vi "Copy Installed VIPM Files to Unpacked Data Folder.vi"(8 "error in (no error)":errorcluster, 9 "LabVIEW version":string, 10 "VIPM Package Installed Filepaths":path[](array[path]), 11 "Unpacked Data Folder":path) -> (0 "error out":errorcluster, 1 "LabVIEW version out":string)   [LabVIEW 2014, in "vipm-to-nipm-package-converter.lvlib"]
doc: "Copies the installed files of the specified VIPM package (.vip) into the corresponding nipkg folder structure\n\nINPUT(S):\n<b>LabVIEW version</b>: Specifies the LabVIEW version for the NIPM package to support (\"14.0\", \"14.0 (64-bit)\", \"18.0\", \"18.0 (64-bit)\", etc)"
uses:
  vipm-to-nipm-package-converter.lvlib
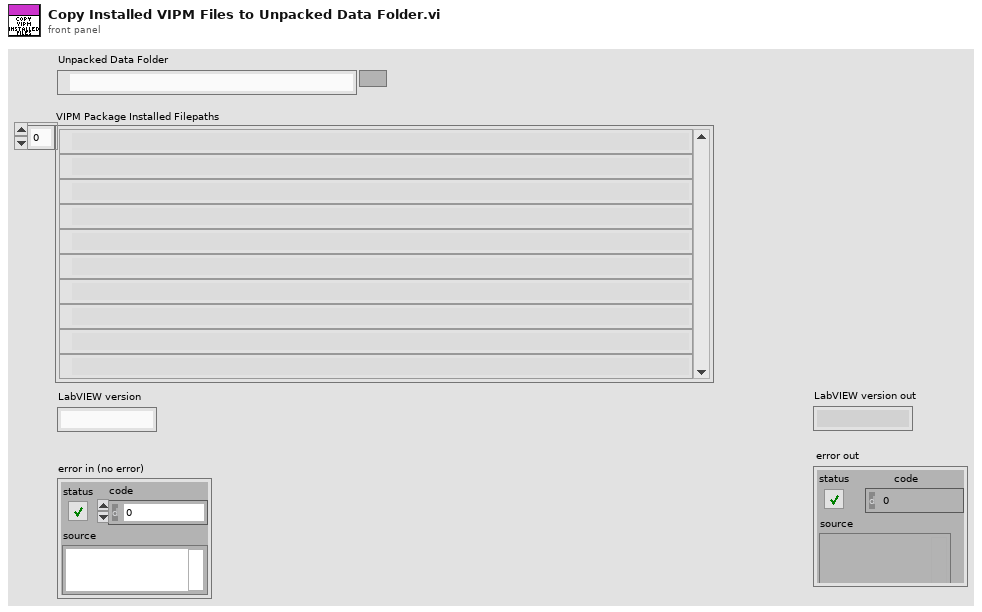
[diagram p1: front panel]
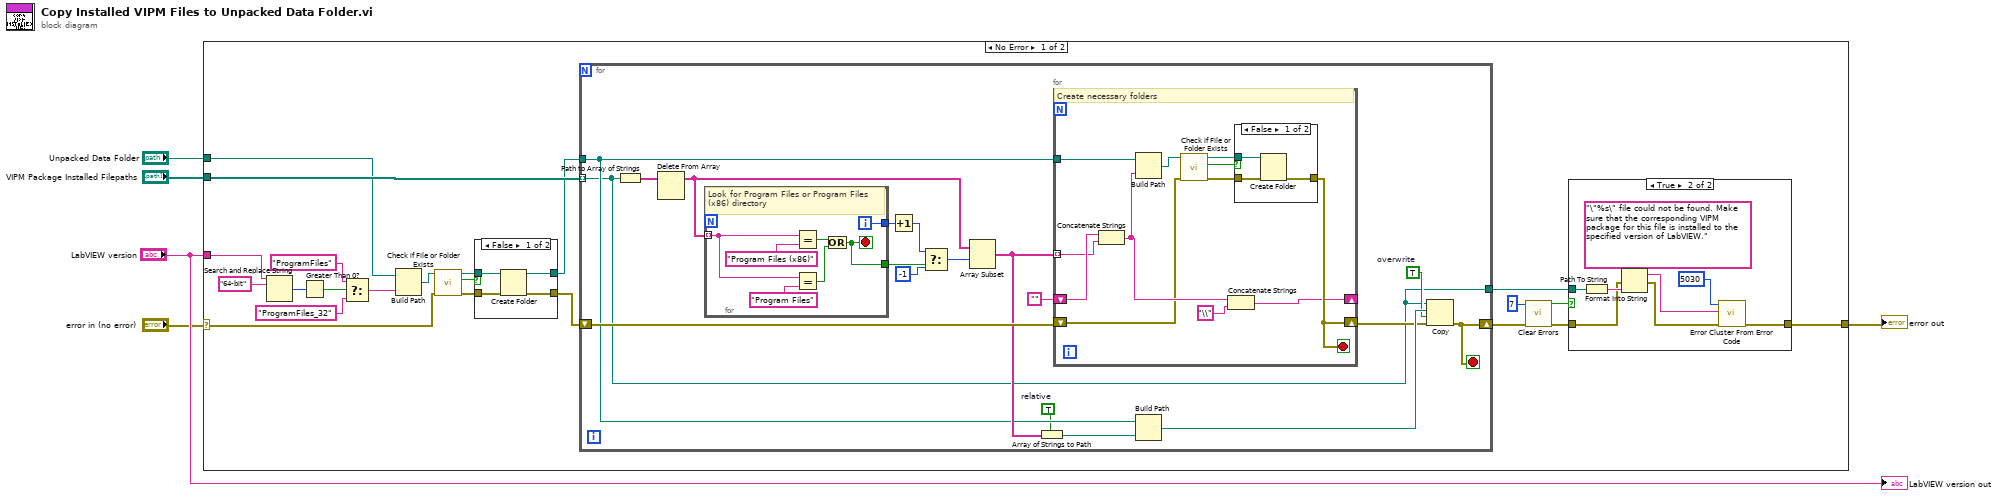
[diagram p0: block diagram]
diagram:
  n1 = case shown="No Error" "error in (no error)" {
    selector: "error in (no error)" -> [w12 w84]
    tunnel: "VIPM Package Installed Filepaths" -> [w27 _]
    tunnel: [w6 w84] -> w4
    tunnel: "Unpacked Data Folder" -> [w22 _]
    tunnel: "LabVIEW version" -> [w13 _]
    frame No Error {
      n2 = Search and Replace String(input string=w13, search string="64-bit") -> (number of replacements=w18:i32)  [unwired: 6 in, 3 out]
      n3 = Greater Than 0?(x=w18) -> (x > 0?=w17:bool)
      n4 = Select(t="ProgramFiles" ("search string"), s=w17, f="ProgramFiles_32" ("search string")) -> (s? t:f=w14:string)
      n5 = Build Path(base path=w22, name or relative path=w14) -> (appended path=w23:path)
      n6 = call <vilib>:"Check if File or Folder Exists.vi"("error in (no error)"=w12, "path"=w23) -> ("error out"=w26:errorcluster, "file or folder exists?"=w24:bool, "dup path"=w25:path)  [unwired: 7 in]
      n7 = case shown="False" w24 {
        tunnel: w25 -> [w40 w41]
        tunnel: w26 -> [w39 w42]
        tunnel: [w38 w42] -> w21
        tunnel: [w37 w41] -> w20
        frame False {
          n8 = Create Folder(path (use dialog)=w40, error in=w39) -> (created path=w37:path, error out=w38:errorcluster)  [unwired: 1 in, 1 out]
        }
        frame True {
        }
      }
      n9 = for {
        tunnel: w27 -> [w43] mode=indexing
        tunnel: w20 -> [w53]
        shift-right: [w54] -> w11
        shift-left: w21 -> [w59]
        tunnel: [w43] -> w7
        stop <- w54 stop-if-true
        w50 = TRUE  # overwrite
        w52 = TRUE  # relative
        n10 = Path to Array of Strings(0:w43) -> (2:w51:string[])  [unwired: 1 out]
        n11 = Delete From Array(array=w51) -> (array with subset deleted=w45:string[])  [unwired: 2 in, 1 out]
        n12 = for {
          tunnel: w45 -> [w66] mode=indexing
          tunnel: [w62] -> w46
          tunnel: [w61] -> w47
          i -> [w61]
          stop <- w62 stop-if-true
          # "Look for Program Files or Program Files (x86) directory"
          n13 = Equal?(x=w66, y="Program Files (x86)") -> (x = y?=w64:bool)
          n14 = Equal?(x=w66, y="Program Files") -> (x = y?=w63:bool)
          n15 = Or(x=w64, y=w63) -> (x .or. y?=w62:bool)
        }
        n16 = Increment(x=w47) -> (x+1=w48:i32)
        n17 = Select(t=w48, s=w46, f=-1) -> (s? t:f=w44:i32)
        n18 = Array Subset(array=w45, index=w44) -> (w58:string[])  [unwired: 1 in]
        n19 = Array of Strings to Path(0:w58, 1:w52) -> (2:w57:path)
        n20 = for {
          tunnel: w53 -> [w79]
          tunnel: w58 -> [w70] mode=indexing
          shift-right: [w69] -> _
          shift-left: "" -> [w74]
          shift-right: [w71] -> w55
          shift-left: w59 -> [w72]
          stop <- w71 stop-if-true
          # "Create necessary folders"
          n21 = Concatenate Strings(w74, w70) -> (w73:string)
          n22 = Build Path(base path=w79, name or relative path=w73) -> (appended path=w78:path)
          n23 = call <vilib>:"Check if File or Folder Exists.vi"("error in (no error)"=w72, "path"=w78) -> ("error out"=w75:errorcluster, "file or folder exists?"=w77:bool, "dup path"=w76:path)  [unwired: 7 in]
          n24 = Concatenate Strings(w73, "\\" ("string")) -> (w69:string)
          n25 = case shown="False" w77 {
            tunnel: w76 -> [w82 _]
            tunnel: w75 -> [w81 w83]
            tunnel: [w80 w83] -> w71
            frame False {
              n26 = Create Folder(path (use dialog)=w82, error in=w81) -> (error out=w80:errorcluster)  [unwired: 1 in, 2 out]
            }
            frame True {
            }
          }
        }
        n27 = Build Path(base path=w53, name or relative path=w57) -> (appended path=w56:path)
        n28 = Copy(8:w55, 9:w50, 10:w56, 11:w43) -> (0:w54:errorcluster)  [unwired: 1 in, 2 out]
      }
      n29 = call <vilib>:"Clear Errors.vi"("error in (no error)"=w11, "specific error code to clear (0: all)"=7) -> ("error out"=w8:errorcluster, "specific error cleared?"=w9:bool)  [unwired: 4 in]
      n30 = case shown="True" w9 {
        tunnel: w8 -> [w28 w32]
        tunnel: w7 -> [_ w34]
        tunnel: [w28 w30] -> w6
        frame False {
        }
        frame True {
          n31 = Path To String(path=w34) -> (string=w33:string)
          n32 = Format Into String(format string="\"%s\" file could not be found. Make sure that the corresponding VIPM package for this file is installed to the specified version of LabVIEW." ("error message (\"\")"), error in=w32, w33) -> (resulting string=w29:string, error out=w31:errorcluster)  [unwired: 1 in]
          n33 = call <vilib>:"Error Cluster From Error Code.vi"("error in (no error)"=w31, "error message (\"\")"=w29, "error code (0)"=5030) -> ("error out"=w30:errorcluster)  [unwired: 6 in]
        }
      }
    }
    frame Error {
    }
  }
  "error out" <- w4
  "LabVIEW version out" <- "LabVIEW version"
